vi "readConfigFileDefault.vi"(8 "error in (no error)":errorcluster) -> (0 "error out":errorcluster, 1 "regTel":string[][](array[string]), 2 "regEvt":string[][](array[string]), 3 "regCmd":string[](array[string]))   [LabVIEW 2018]
doc: "Read the default.ini file to get commands, events and telemetry that will be registered by TCP Server."
uses:
  <vilib>/Utility/config.llb/NI_LVConfig.lvlib
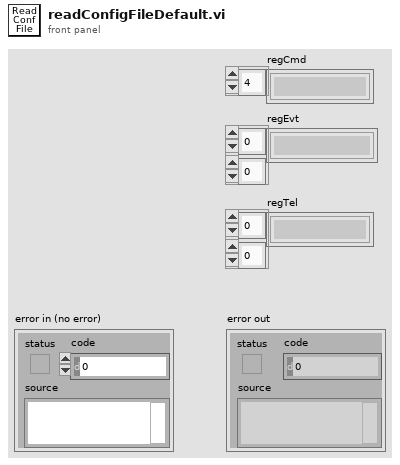
[diagram p1: front panel]
types:
  T1 = typedef "NI_LVConfig.lvlib/Config Data RefNum.ctl" = refnum<k1>
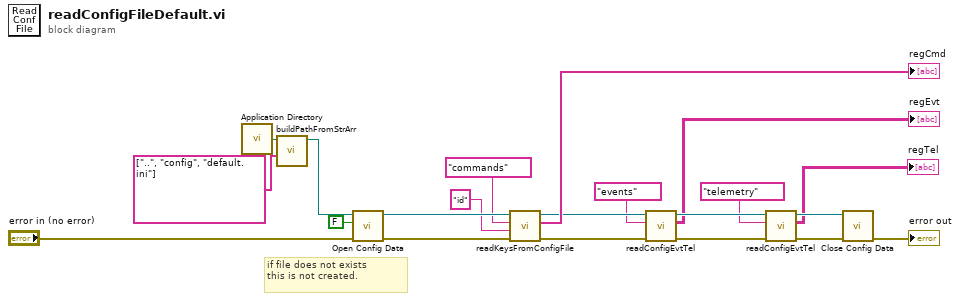
[diagram p0: block diagram]
diagram:
  # "if file does not exists\nthis is not created."
  n1 = call <vilib>:"Application Directory.vi"() -> ("Application Directory"=w13:path)
  n2 = call "buildPathFromStrArr.vi"("String Array"=string[] ["..", "config", "default.ini"], "Root Path"=w13) -> ("Absolute Path"=w11:path)  [unwired: 9 in]
  n3 = call <vilib>:"Open Config Data.vi"("error in (no error)"="error in (no error)", "create file if necessary (T)"=FALSE, "configuration file path"=w11) -> ("error out"=w8:errorcluster, "refnum"=w9:T1)  [unwired: 6 in, 1 out]
  n4 = call "readKeysFromConfigFile.vi"("error in (no error)"=w8, "key"="id", "section"="commands", "Refnum in"=w9) -> ("error out"=w19:errorcluster, "arrayOfKeys"=→"regCmd":string[], "Refnum out"=w20:T1)  [unwired: 5 in]
  n5 = call "readConfigEvtTel.vi"("error in (no error)"=w19, "item"="events", "Path in"=w20) -> ("error out"=w18:errorcluster, "regEvt/Tel"=→"regEvt":string[][], "Path out"=w17:T1)  [unwired: 6 in]
  n6 = call "readConfigEvtTel.vi"("error in (no error)"=w18, "item"="telemetry", "Path in"=w17) -> ("error out"=w14:errorcluster, "regEvt/Tel"=→"regTel":string[][], "Path out"=w16:T1)  [unwired: 6 in]
  n7 = call <vilib>:"Close Config Data.vi"("error in (no error)"=w14, "refnum"=w16) -> ("error out"=→"error out":errorcluster)  [unwired: 8 in, 1 out]
